vi "Set Visible State on Multiple Controls.vi"(10 "Visible?":bool, 11 "Controls":refnum<vi>[](array[refnum])) -> ()   [LabVIEW 2016, in "Common.lvlib"]
doc: "Sets all the controls in the input array to the \"Enable state\" value."
uses:
  <userlib>/Common Components/Common/Common.lvlib
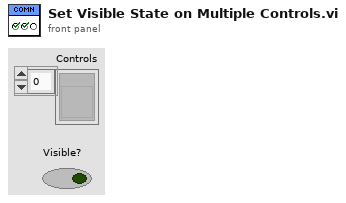
[diagram p1: front panel]
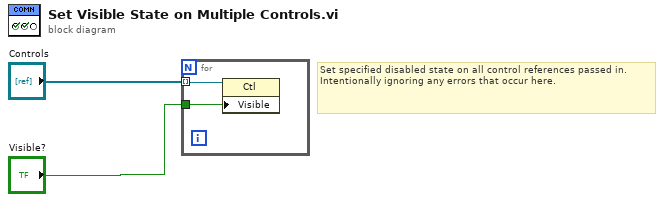
[diagram p0: block diagram]
diagram:
  # "Set specified disabled state on all control references passed in. Intentionally ignoring any errors that occur here."
  n1 = for {
    tunnel: "Controls" -> [w4] mode=indexing
    tunnel: "Visible?" -> [w3]
    n2 = property class="Ctl"(reference=w4, "Visible"=w3) -> ()  [unwired: 1 in, 2 out]
  }
